vi "Parse_DevBuffer.vi"(8 "error in (no error)":errorcluster, 10 "searchFor":string, 11 "Multiplexer_Opmux in":refnum<class "Multiplexer_Opmux.lvclass">) -> (0 "error out":errorcluster, 2 "Found":bool, 3 "Multiplexer_Opmux out":refnum<class "Multiplexer_Opmux.lvclass">)   [LabVIEW 2013, in "Multiplexer_Opmux.lvclass"]
uses:
  Multiplexer_Opmux.lvclass
  Multiplexer_Opmux.lvclass/Multiplexer_Opmux.ctl
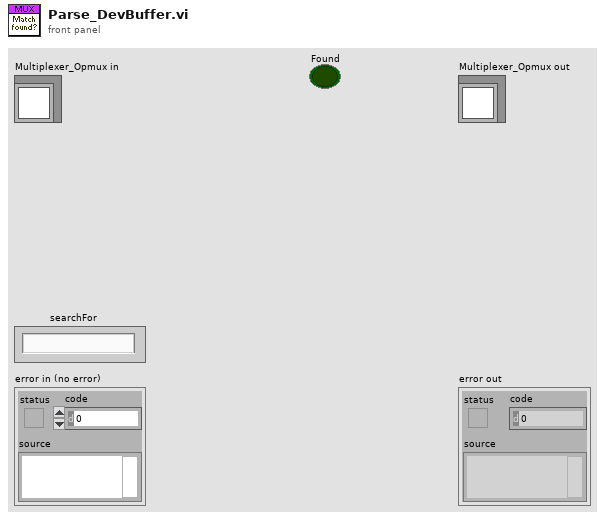
[diagram p1: front panel]
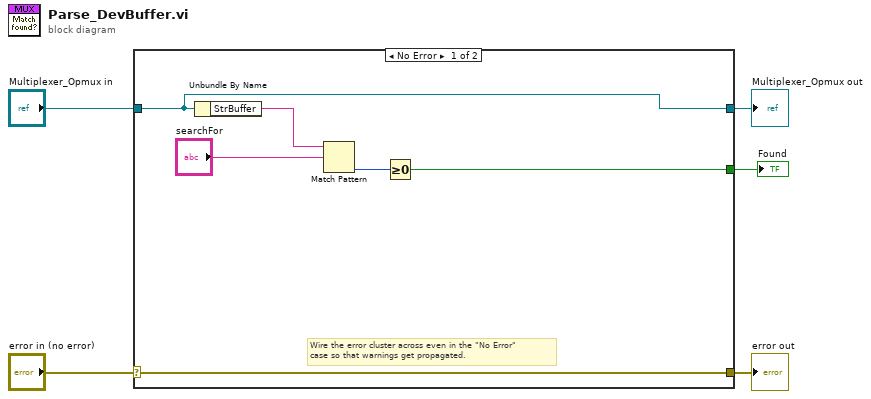
[diagram p0: block diagram]
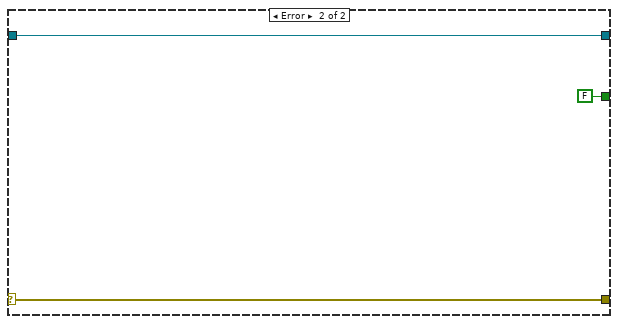
[diagram p2: hidden frame]
diagram:
  n1 = case shown="No Error" "error in (no error)" {
    selector: "error in (no error)" -> [w11 w14]
    tunnel: [w11 w14] -> w4
    tunnel: [w8 w13] -> w2
    tunnel: "Multiplexer_Opmux in" -> [w8 w13]
    tunnel: [w6 FALSE] -> w1
    frame No Error {
      # "Wire the error cluster across even in the \"No Error\"\ncase so that warnings get propagated."
      n2 = Unbundle By Name(w8) -> ("StrBuffer"=w9:string)
      n3 = Match Pattern(string=w9, regular expression="searchFor") -> (offset past match=w7:i32)  [unwired: 1 in, 3 out]
      n4 = Greater Or Equal To 0?(x=w7) -> (x >= 0?=w6:bool)
    }
    frame Error {
    }
  }
  "error out" <- w4
  "Multiplexer_Opmux out" <- w2
  "Found" <- w1
